vi "Timer FGV.vi"(7 "Timer Action":T1, 8 "error in (no error)":errorcluster, 11 "Target Time":dbl) -> (0 "error out":errorcluster, 2 "Elapsed ?":bool, 3 "Elapsed Time":dbl)   [LabVIEW 2017]
doc: "Pausable FGV Timer"
uses:
  Controls/Timer - Action.ctl
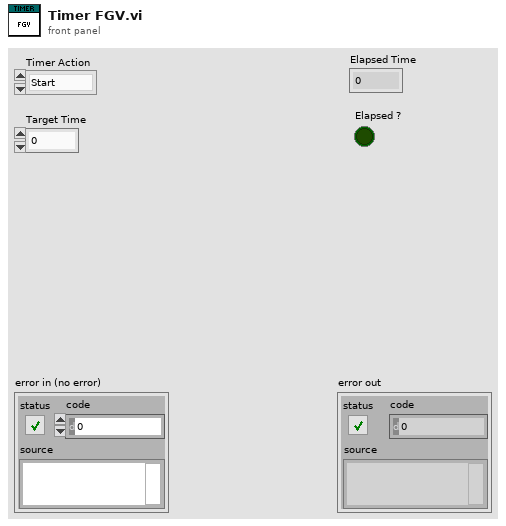
[diagram p1: front panel]
types:
  T1 = typedef "Timer - Action.ctl" = enum16{"Start", "Get Time", "Pause", "UnPause"}
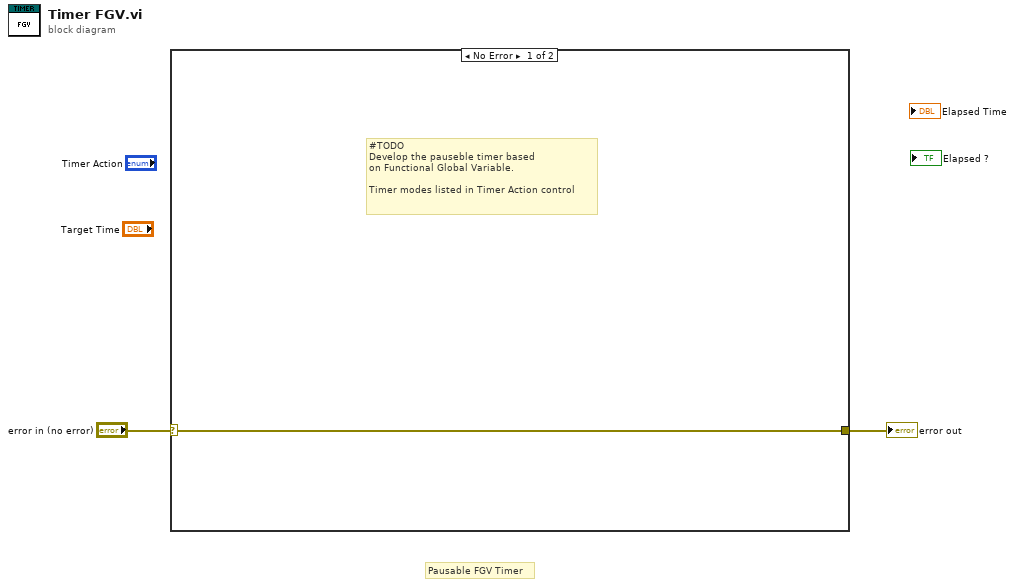
[diagram p0: block diagram]
diagram:
  # "Pausable FGV Timer"
  n1 = case shown="No Error" "error in (no error)" {
    selector: "error in (no error)" -> [w3 w4]
    tunnel: [w3 w4] -> w1
    frame No Error {
      # "#TODO\nDevelop the pauseble timer based\non Functional Global Variable.\n\nTimer modes listed in Timer Action control"
    }
    frame Error {
    }
  }
  "error out" <- w1
